vi "Fit EPR Spectra_Rev5.vi"(0 "Spectral Data In":T2={"PDT Amp [v]"=0.0, "RIS Amp [v]"=0.0, "B-Field"=[], "All In-Phase Scan Spectra"=[], "Model Select"=enum."OneCompRISTwoPDT", "Fit Each Scan"=FALSE, "PDT Center [g]"=0.0, "In-Phase Average Spectra"=[], "In-Phase Median Spectra"=[], "Out-Phase Median Spectra"=[], "Out-Phase Average Spectra"=[], "Fit Spectra"=[], "Fit No-Baseline Spectra"=[], "All Out-Phase Scan Spectra"=[], "Baseline Offset Correction"=FALSE, "In-Phase Offset [v]"=0.0, "Out-Phase Offset [v]"=0.0, "Ch2 Input\n(Balance)"=[], "Ch3 Input\n(Phase)"=[], "Ch4 Input\n(AFC)"=[], "Fit Pars"=[], "Fit Pars Errors"=[], "Fit Pars Labels"=[], "Raw Scan DAQ Data"=[], "Bad Scans Indicies"=[], "Good In-Phase Scan Spectra"=[], "Good Out-Phase Scan Spectra"=[], "Bad In-Phase Scan Spectra"=[], "Bad Out-Phase Scan Spectra"=[], "Number of bad scans"=0, "Fit History"=[], "PDT Amp. History/Set [v]"=[], "RIS Amp. History/Set [v]"=[], "RIS Amp. History/Scan [v]"=[], "All Shifted B-Fields"=[], "Good Shifted B-Fields"=[], "Ch5 Input\n(SpO2)"=[], "Ch6 Input\n(BPM)"=[], "Global SNR"=0.0, "Fit Error History"=[], "SNR History"=[]} {"Global SNR" min=0.0; "PDT Center [g]" min=0.0; "RIS Amp [v]" min=0.0}, 5 "B":dbl[](array[numeric])=array[4097 elements], 9 "y":dbl[](array[numeric])=array[4097 elements], 11 "modFreq":dbl, 12 "modAmp":dbl) -> (1 "fitNoBaseline":dbl[](array[numeric]), 3 "pars":dbl[](array[numeric]), 4 "parsError":dbl[](array[numeric]), 6 "vpp":dbl[](array[numeric]), 10 "fit":dbl[](array[numeric]), 13 "Global SNR":dbl, 14 "error out":errorcluster, 15 "Number of Fit Iterations":i32)   [LabVIEW 2016]
uses:
  EPR DAQ/qsm/trunk/Types/Spectral Data.ctl
  EPR DAQ/qsm/trunk/Types/Fitting Model Selection.ctl
  <vilib>/Analysis/NI_AALBase.lvlib
  <vilib>/Analysis/NI_AALPro.lvlib
  Rev5/libFitSpectraLabview_Rev5.lvlib
panel:
  out "Model Select":T1=enum."OneCompRISTwoPDT"
  in  "model":u16(ring) items=["OneCompRIS", "OneCompRISRev", "OneCompRISTwoPDT", "OneCompRISTwoPDTRev", "LiPc", "TwoLiPc", "ThreeLiPc", "FourLiPc", "PDTCalibration", "CE_Ink", "Printex"]
  out "noise":dbl
  out "snr":dbl[](array[numeric])
  # "See model choices."
  # "Magnetic Field [G]"
  # "Signal [AU]"
  # "Parameters\n1. Modulation Frequency [G]\n2. Modulation Amplitude [G]\n3. Phase [rad]\n4. Baseline offet [AU]\n5. Baseline slope [AU/G]\n6+3*N. Center [G]\n7+3*N. Linewidth (HWHM) [G]\n8+3*N. Intensity [AU]\n\nwhere N is the component number, \nindexed from 0. Components are\nlisted from high-field to low-field."
  # "Model Choices\n1. OneCompRIS - Tooth Dosimetry, high-field PDT with tooth signal 10.3 G down-field; the tooth is fit to a single component\n      for the radiation-induced signal (RIS), instead of separate components for the native signal and the radiation-induced signal.\n2. OneCompRISRev - same as above, but with 12.3 G separation between the PDT and tooth signal; for reverse polarity measurements.\n3. OneCompRISTwoPDT - Same as above, except that both the low-field and high-field PDTs are included. The low-field PDT is\n      locked to the high-field PDT, such that they are forced to have identical spectral parameters.\n4. OneCompRISTwoPDTRev - Same as above, but with 12.3 G separation between the PDT and tooth signals; for reverse polarity\n      measurements.\n5. LiPc - Oximetry, single LiPc component, modulation amplitude and phase are both fixed.\n6. TwoLiPc - same as above, but with two LiPc components.\n7. ThreeLiPc - same as above, but with three LiPc components.\n8. FourLiPc - same as above, but with four LiPc components.\n9. PDTCalibration - high-field and low-field PDT components with variable centers\n10. CE_Ink - Carlo Erba Ink: Locked centers, fixed relationship from LW1 to LW2, and INT1 to INT2\n11. Printex - 2 LiPc components with locked centers"
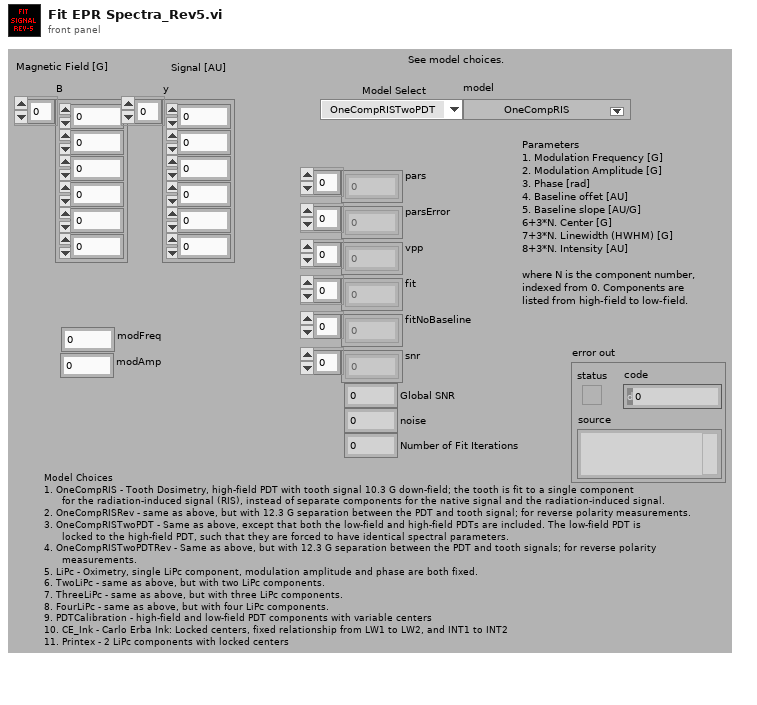
[diagram p1: front panel]
types:
  T1 = typedef "Fitting Model Selection.ctl" = enum16{"OneCompRIS", "OneCompRISTwoPDT", "OneCompRISRev", "OneCompRISTwoPDTRev", "LiPc", "TwoLiPc", "ThreeLiPc", "FourLiPc", "PDTCalibration", "CE_Ink", "Printex", "MelaninTwoPDT"}
  T2 = typedef "Spectral Data.ctl" = cluster{"PDT Amp [v]":dbl, "RIS Amp [v]":dbl, "B-Field":dbl[], "All In-Phase Scan Spectra":dbl[][], "Model Select":T1, "Fit Each Scan":bool, "PDT Center [g]":dbl, "In-Phase Average Spectra":dbl[], "In-Phase Median Spectra":dbl[], "Out-Phase Median Spectra":dbl[], "Out-Phase Average Spectra":dbl[], "Fit Spectra":dbl[], "Fit No-Baseline Spectra":dbl[], "All Out-Phase Scan Spectra":dbl[][], "Baseline Offset Correction":bool, "In-Phase Offset [v]":dbl, "Out-Phase Offset [v]":dbl, "Ch2 Input\n(Balance)":dbl[], "Ch3 Input\n(Phase)":dbl[], "Ch4 Input\n(AFC)":dbl[], "Fit Pars":dbl[], "Fit Pars Errors":dbl[], "Fit Pars Labels":string[], "Raw Scan DAQ Data":dbl[][], "Bad Scans Indicies":i32[], "Good In-Phase Scan Spectra":dbl[][], "Good Out-Phase Scan Spectra":dbl[][], "Bad In-Phase Scan Spectra":dbl[][], "Bad Out-Phase Scan Spectra":dbl[][], "Number of bad scans":i32, "Fit History":dbl[][], "PDT Amp. History/Set [v]":dbl[], "RIS Amp. History/Set [v]":dbl[], "RIS Amp. History/Scan [v]":dbl[], "All Shifted B-Fields":dbl[][], "Good Shifted B-Fields":dbl[][], "Ch5 Input\n(SpO2)":dbl[], "Ch6 Input\n(BPM)":dbl[], "Global SNR":dbl, "Fit Error History":dbl[][], "SNR History":dbl[]}
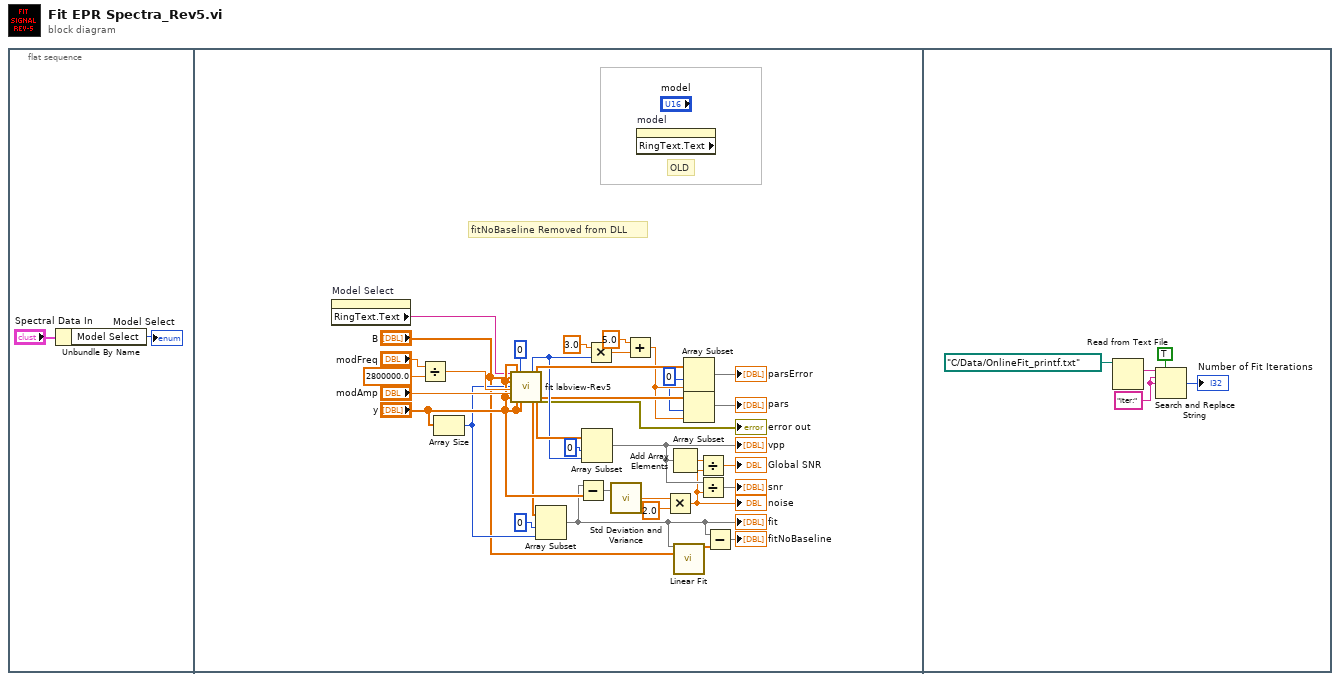
[diagram p0: block diagram]
diagram:
  n1 = flat-sequence {
    frame #0 {
      n2 = Unbundle By Name("Spectral Data In") -> ("Model Select"=→"Model Select":T1)
    }
    frame #1 {
      w10 = 0 ("index")
      # "fitNoBaseline Removed from DLL"
      # "OLD"
      n3 = property on="Model Select" class="Enum (strict)"() -> ("RingText.Text"=w14:string)  [unwired: 2 in, 2 out]
      n4 = Divide(x="modFreq", y=2800000.0) -> (x/y=w31:dbl)
      n5 = Array Size(array="y") -> (size(s)=w15:i32)
      n6 = call "fit labview-Rev5.vi"("modelname"=w14, "B"="B", "y"="y", "npts"=w15, "modFreq"=w31, "modAmp"="modAmp", "pars"="y", "parsError"="y", "vpp"="y", "ncomps"=0, "fit"="y") -> ("ncomps out"=w27:i32, "fit out"=w17:dbl[], "parsError out"=w30:dbl[], "vpp out"=w28:dbl[], "pars out"=w25:dbl[], "error out"=→"error out":errorcluster)  [unwired: 11 in]
      n7 = Array Subset(array=w17, index=0, length=w15) -> (w8:dbl[])
      "fit" <- w8
      n8 = Subtract(x=w8, y="y") -> (x-y=w19:dbl[])
      n9 = Array Subset(array=w28, index=0, length=w27) -> (w6:dbl[])
      "vpp" <- w6
      n10 = Multiply(x=3.0, y=w27) -> (x*y=w36:dbl)
      n11 = call <vilib>:"Std Deviation and Variance.vi"("X"=w19) -> ("standard deviation"=w18:dbl)  [unwired: 1 in, 2 out]
      n12 = Add(x=5.0, y=w36) -> (x+y=w24:dbl)
      n13 = property on="model" class="Ring (strict)" props=["RingText", "Text"]() -> ()  [unwired: 2 in, 3 out]
      n14 = Multiply(x=w18, y=2.0) -> (x*y=w4:dbl)
      "noise" <- w4
      n15 = Add Array Elements(numeric array=w6) -> (sum=w5:dbl)
      n16 = call <vilib>:"Linear Fit.vi"("Y"=w8, "X"="B") -> ("Best Linear Fit"=w11:dbl[])  [unwired: 9 in, 4 out]
      n17 = Array Subset(array=w30, index=w10, length=w24) -> (→"parsError":dbl[])
      n18 = Array Subset(array=w25, index=w10, length=w24) -> (→"pars":dbl[])
      n19 = Divide(x=w5, y=w4) -> (x/y=→"Global SNR":dbl)
      n20 = Divide(x=w6, y=w4) -> (x/y=→"snr":dbl[])
      n21 = Subtract(x=w8, y=w11) -> (x-y=→"fitNoBaseline":dbl[])
    }
    frame #2 {
      w40 = "iter:" ("search string")
      n22 = Read from Text File(file (use dialog)=path "C:/Data/OnlineFit_printf.txt") -> (text=w41:string)  [unwired: 3 in, 3 out]
      n23 = Search and Replace String(replace all?=TRUE ("replace all? (F)"), input string=w41, search string=w40, replace string=w40) -> (number of replacements=→"Number of Fit Iterations":i32)  [unwired: 4 in, 3 out]
    }
  }
